vi "pcfs_initialize_detector.vi"(8 "error in (no error)":errorcluster, 11 "pcfs in":refnum<class "pcfs.lvclass">) -> (0 "error out":errorcluster, 3 "pcfs out":refnum<class "pcfs.lvclass">)   [LabVIEW 2015, in "pcfs.lvclass"]
uses:
  pcfs.lvclass
  UI/front_panel_class/hardware_caller_queue_numbers.ctl
  Detector_Class/detector/detector.lvclass
  pcfs.lvclass/pcfs.ctl
  UI/panel_class/panel.lvclass
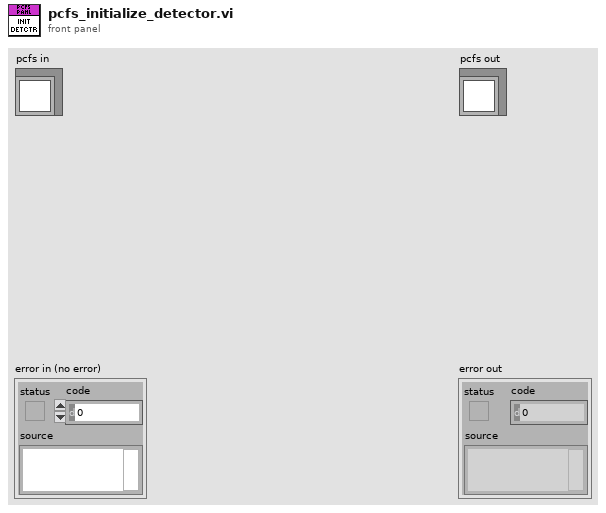
[diagram p1: front panel]
types:
  T1 = typedef "hardware_caller_queue_numbers.ctl" = enum16{"stage1", "stage2", "experiment", "detector"}
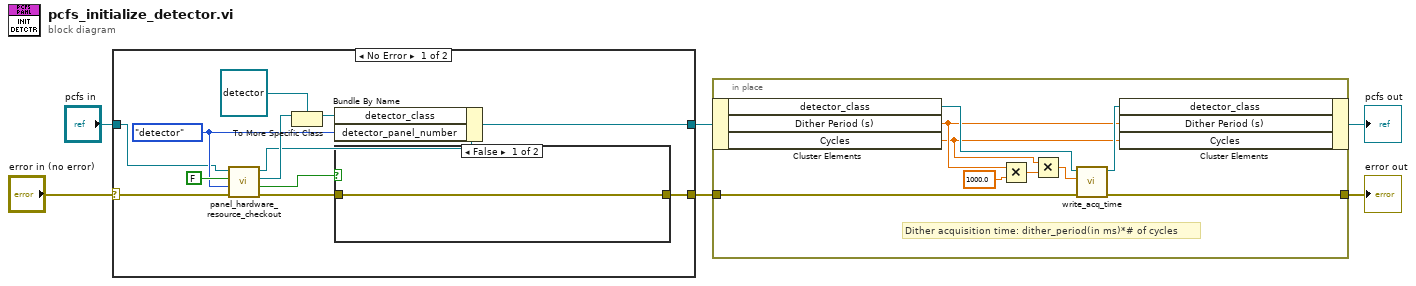
[diagram p0: block diagram]
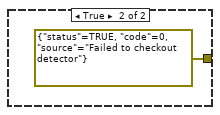
[diagram p2: hidden frame]
diagram:
  n1 = case shown="No Error" "error in (no error)" {
    selector: "error in (no error)" -> [w16 w22]
    tunnel: [w13 w22] -> w1
    tunnel: [w14 w21] -> w4
    tunnel: "pcfs in" -> [w11 w21]
    frame No Error {
      w12 = hardware_caller_queue_numbers."detector" ("panel_number")
      n2 = call "panel_hardware_resource_checkout.vi"("error in (no error)"=w16, "panel_number"=w12, "Self?"=FALSE, "panel in"=w11) -> ("error out"=w8:errorcluster, "timed out?"=w7:bool, "hardware.lvclass"=w15:refnum<class "hardware.lvclass">, "panel out"=w10:refnum<class "pcfs.lvclass">)  [unwired: 4 in]
      n3 = To More Specific Class(target class=refnum<class "detector.lvclass"> refnum ("detector.lvclass"), reference=w15) -> (specific class reference=w9:refnum<class "detector.lvclass">)  [unwired: 1 in, 1 out]
      n4 = Bundle By Name(cluster=w10, "detector_class"=w9, "detector_panel_number"=w12) -> (w14:refnum<class "pcfs.lvclass">)
      n5 = case shown="False" w7 {
        tunnel: [w19 errorcluster {"status"=TRUE, "code"=0, "source"="Failed to checkout detector"} ("error out")] -> w13
        tunnel: w8 -> [w19 _]
        frame False {
        }
        frame True {
        }
      }
    }
    frame Error {
    }
  }
  n6 = in-place {
    in-place-border: [w29] -> w2
    in-place-border: w1 -> [w28]
    # "Dither acquisition time: dither_period(in ms)*# of cycles"
    n7 = in-place-cluster #1(w4) -> ("detector_class"=w27:refnum<class "detector.lvclass">, "Dither Period (s)"=w25:dbl, "Cycles"=w23:dbl)
    n8 = Multiply(x=w25, y=1000.0) -> (x*y=w24:dbl)
    n9 = Multiply(x=w23, y=w24) -> (x*y=w30:dbl)
    n10 = call-dynamic "write_acq_time.vi"("error in (no error)"=w28, "acq_time"=w30, "detector in"=w27) -> ("error out"=w29:errorcluster, "detector out"=w26:refnum<class "detector.lvclass">)  [unwired: 7 in]
    n11 = in-place-cluster #1("detector_class"=w26, "Dither Period (s)"=w25, "Cycles"=w23) -> (→"pcfs out":refnum<class "pcfs.lvclass">)
  }
  "error out" <- w2
